vi "Register gRPC Messages.vi"(8 "error in (no error)":errorcluster, 11 "gRPC ID":T1) -> (0 "error out":errorcluster, 3 "gRPC ID Out":T1)   [LabVIEW 2021, in "NI Switch Client.lvlib"]
uses:
  NI Switch Client.lvlib
  <vilib>/gRPC/LabVIEW gRPC Library/Shared/grpcId.ctl
  <vilib>/gRPC/LabVIEW gRPC Library/Server API/typeDefs/Message Metadata.ctl
  <vilib>/gRPC/LabVIEW gRPC Library/Server API/typeDefs/Message Element Metadata.ctl
  <vilib>/gRPC/LabVIEW gRPC Library/Server API/typeDefs/Message Element Type.ctl
  <vilib>/gRPC/LabVIEW gRPC Library/Server API/typeDefs/Enum Metadata.ctl
  <vilib>/gRPC/LabVIEW gRPC Library/grpc-lvsupport-release.lvlib
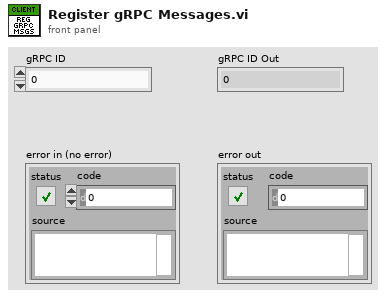
[diagram p1: front panel]
types:
  T1 = typedef "grpc-lvsupport-release.lvlib/grpcId.ctl" = u64
  T2 = typedef "grpc-lvsupport-release.lvlib/Enum Metadata.ctl" = cluster{"Version":i32, "Name":string, "Type Url":string, "Enum Values":string, "Allow Alias":bool}
  T3 = typedef "grpc-lvsupport-release.lvlib/Message Metadata.ctl" = cluster{"Version":i32, "Name":string, "Type Url":string, "Elements":T4[], "Has Oneof":bool}
  T4 = typedef "grpc-lvsupport-release.lvlib/Message Element Metadata.ctl" = cluster{"Field Name":string, "Embedded Message Name":string, "Protobuf Index":i32, "MessageElementType":T5, "Repeated":bool, "Is in Oneof":bool, "Oneof Container Name":string}
  T5 = typedef "grpc-lvsupport-release.lvlib/Message Element Type.ctl" = enum32{"Int32Value", "FloatValue", "DoubleValue", "BoolValue", "StringValue", "MessageValue", "Int64Value", "UInt32Value", "UInt64Value", "EnumValue", "Bytes", "Fixed64", "Fixed32", "SFixed64", "SFixed32", "SInt64", "SInt32"}
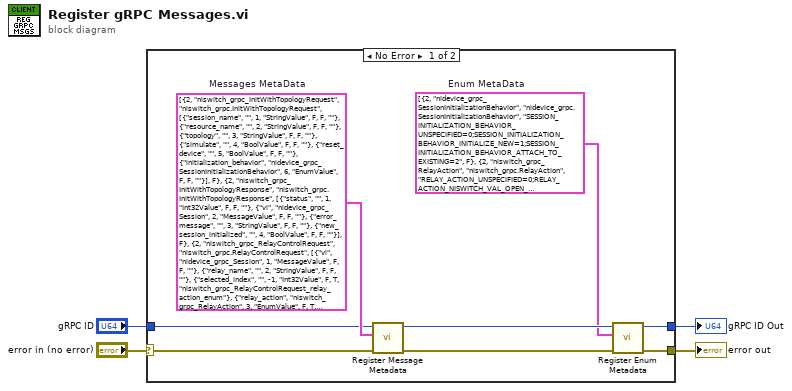
[diagram p0: block diagram]
diagram:
  n1 = case shown="No Error" "error in (no error)" {
    selector: "error in (no error)" -> [w10 w13]
    tunnel: [w9 w12] -> w1
    tunnel: [w6 w13] -> w4
    tunnel: "gRPC ID" -> [w9 w12]
    frame No Error {
      w5 = T2[] [{"Version"=2, "Name"="nidevice_grpc_SessionInitializationBehavior", "Type Url"="nidevice_grpc.SessionInitializationBehavior", "Enum Values"="SESSION_INITIALIZATION_BEHAVIOR_UNSPECIFIED=0;SESSION_INITIALIZATION_BEHAVIOR_INITIALIZE_NEW=1;SESSION_INITIALIZATION_BEHAVIOR_ATTACH_TO_EXISTING=2", "Allow Alias"=FALSE}, {"Version"=2, "Name"="niswitch_grpc_RelayAction", "Type Url"="niswitch_grpc.RelayAction", "Enum Values"="RELAY_ACTION_UNSPECIFIED=0;RELAY_ACTION_NISWITCH_VAL_OPEN_RELAY=20;RELAY_ACTION_NISWITCH_VAL_CLOSE_RELAY=21", "Allow Alias"=FALSE}, {"Version"=2, "Name"="niswitch_grpc_RelayPosition", "Type Url"="niswitch_grpc.RelayPosition", "Enum Values"="RELAY_POSITION_UNSPECIFIED=0;RELAY_POSITION_NISWITCH_VAL_OPEN=10;RELAY_POSITION_NISWITCH_VAL_CLOSED=11", "Allow Alias"=FALSE}]  # Enum MetaData
      w11 = T3[] [{"Version"=2, "Name"="niswitch_grpc_InitWithTopologyRequest", "Type Url"="niswitch_grpc.InitWithTopologyRequest", "Elements"=[{"Field Name"="session_name", "Embedded Message Name"="", "Protobuf Index"=1, "MessageElementType"=enum."StringValue", "Repeated"=FALSE, "Is in Oneof"=FALSE, "Oneof Container Name"=""}, {"Field Name"="resource_name", "Embedded Message Name"="", "Protobuf Index"=2, "MessageElementType"=enum."StringValue", "Repeated"=FALSE, "Is in Oneof"=FALSE, "Oneof Container Name"=""}, {"Field Name"="topology", "Embedded Message Name"="", "Protobuf Index"=3, "MessageElementType"=enum."StringValue", "Repeated"=FALSE, "Is in Oneof"=FALSE, "Oneof Container Name"=""}, {"Field Name"="simulate", "Embedded Message Name"="", "Protobuf Index"=4, "MessageElementType"=enum."BoolValue", "Repeated"=FALSE, "Is in Oneof"=FALSE, "Oneof Container Name"=""}, {"Field Name"="reset_device", "Embedded Message Name"="", "Protobuf Index"=5, "MessageElementType"=enum."BoolValue", "Repeated"=FALSE, "Is in Oneof"=FALSE, "Oneof Container Name"=""}, {"Field Name"="initialization_behavior", "Embedded Message Name"="nidevice_grpc_SessionInitializationBehavior", "Protobuf Index"=6, "MessageElementType"=enum."EnumValue", "Repeated"=FALSE, "Is in Oneof"=FALSE, "Oneof Container Name"=""}], "Has Oneof"=FALSE}, {"Version"=2, "Name"="niswitch_grpc_InitWithTopologyResponse", "Type Url"="niswitch_grpc.InitWithTopologyResponse", "Elements"=[{"Field Name"="status", "Embedded Message Name"="", "Protobuf Index"=1, "MessageElementType"=enum."Int32Value", "Repeated"=FALSE, "Is in Oneof"=FALSE, "Oneof Container Name"=""}, {"Field Name"="vi", "Embedded Message Name"="nidevice_grpc_Session", "Protobuf Index"=2, "MessageElementType"=enum."MessageValue", "Repeated"=FALSE, "Is in Oneof"=FALSE, "Oneof Container Name"=""}, {"Field Name"="error_message", "Embedded Message Name"="", "Protobuf Index"=3, "MessageElementType"=enum."StringValue", "Repeated"=FALSE, "Is in Oneof"=FALSE, "Oneof Container Name"=""}, {"Field Name"="new_session_initialized", "Embedded Message Name"="", "Protobuf Index"=4, "MessageElementType"=enum."BoolValue", "Repeated"=FALSE, "Is in Oneof"=FALSE, "Oneof Container Name"=""}], "Has Oneof"=FALSE}, {"Version"=2, "Name"="niswitch_grpc_RelayControlRequest", "Type Url"="niswitch_grpc.RelayControlRequest", "Elements"=[{"Field Name"="vi", "Embedded Message Name"="nidevice_grpc_Session", "Protobuf Index"=1, "MessageElementType"=enum."MessageValue", "Repeated"=FALSE, "Is in Oneof"=FALSE, "Oneof Container Name"=""}, {"Field Name"="relay_name", "Embedded Message Name"="", "Protobuf Index"=2, "MessageElementType"=enum."StringValue", "Repeated"=FALSE, "Is in Oneof"=FALSE, "Oneof Container Name"=""}, {"Field Name"="selected_index", "Embedded Message Name"="", "Protobuf Index"=-1, "MessageElementType"=enum."Int32Value", "Repeated"=FALSE, "Is in Oneof"=TRUE, "Oneof Container Name"="niswitch_grpc_RelayControlRequest_relay_action_enum"}, {"Field Name"="relay_action", "Embedded Message Name"="niswitch_grpc_RelayAction", "Protobuf Index"=3, "MessageElementType"=enum."EnumValue", "Repeated"=FALSE, "Is in Oneof"=TRUE, "Oneof Container Name"="niswitch_grpc_RelayControlRequest_relay_action_enum"}, {"Field Name"="relay_action_raw", "Embedded Message Name"="", "Protobuf Index"=4, "MessageElementType"=enum."SInt32", "Repeated"=FALSE, "Is in Oneof"=TRUE, "Oneof Container Name"="niswitch_grpc_RelayControlRequest_relay_action_enum"}], "Has Oneof"=TRUE}, {"Version"=2, "Name"="niswitch_grpc_RelayControlResponse", "Type Url"="niswitch_grpc.RelayControlResponse", "Elements"=[{"Field Name"="status", "Embedded Message Name"="", "Protobuf Index"=1, "MessageElementType"=enum."Int32Value", "Repeated"=FALSE, "Is in Oneof"=FALSE, "Oneof Container Name"=""}], "Has Oneof"=FALSE}, {"Version"=2, "Name"="niswitch_grpc_GetRelayPositionRequest", "Type Url"="niswitch_grpc.GetRelayPositionRequest", "Elements"=[{"Field Name"="vi", "Embedded Message Name"="nidevice_grpc_Session", "Protobuf Index"=1, "MessageElementType"=enum."MessageValue", "Repeated"=FALSE, "Is in Oneof"=FALSE, "Oneof Container Name"=""}, {"Field Name"="relay_name", "Embedded Message Name"="", "Protobuf Index"=2, "MessageElementType"=enum."StringValue", "Repeated"=FALSE, "Is in Oneof"=FALSE, "Oneof Container Name"=""}], "Has Oneof"=FALSE}, {"Version"=2, "Name"="niswitch_grpc_GetRelayPositionResponse", "Type Url"="niswitch_grpc.GetRelayPositionResponse", "Elements"=[{"Field Name"="status", "Embedded Message Name"="", "Protobuf Index"=1, "MessageElementType"=enum."Int32Value", "Repeated"=FALSE, "Is in Oneof"=FALSE, "Oneof Container Name"=""}, {"Field Name"="relay_position", "Embedded Message Name"="niswitch_grpc_RelayPosition", "Protobuf Index"=2, "MessageElementType"=enum."EnumValue", "Repeated"=FALSE, "Is in Oneof"=FALSE, "Oneof Container Name"=""}, {"Field Name"="relay_position_raw", "Embedded Message Name"="", "Protobuf Index"=3, "MessageElementType"=enum."SInt32", "Repeated"=FALSE, "Is in Oneof"=FALSE, "Oneof Container Name"=""}], "Has Oneof"=FALSE}, {"Version"=2, "Name"="niswitch_grpc_WaitForDebounceRequest", "Type Url"="niswitch_grpc.WaitForDebounceRequest", "Elements"=[{"Field Name"="vi", "Embedded Message Name"="nidevice_grpc_Session", "Protobuf Index"=1, "MessageElementType"=enum."MessageValue", "Repeated"=FALSE, "Is in Oneof"=FALSE, "Oneof Container Name"=""}, {"Field Name"="maximum_time_ms", "Embedded Message Name"="", "Protobuf Index"=2, "MessageElementType"=enum."SInt32", "Repeated"=FALSE, "Is in Oneof"=FALSE, "Oneof Container Name"=""}], "Has Oneof"=FALSE}, {"Version"=2, "Name"="niswitch_grpc_WaitForDebounceResponse", "Type Url"="niswitch_grpc.WaitForDebounceResponse", "Elements"=[{"Field Name"="status", "Embedded Message Name"="", "Protobuf Index"=1, "MessageElementType"=enum."Int32Value", "Repeated"=FALSE, "Is in Oneof"=FALSE, "Oneof Container Name"=""}], "Has Oneof"=FALSE}, {"Version"=2, "Name"="niswitch_grpc_CloseRequest", "Type Url"="niswitch_grpc.CloseRequest", "Elements"=[{"Field Name"="vi", "Embedded Message Name"="nidevice_grpc_Session", "Protobuf Index"=1, "MessageElementType"=enum."MessageValue", "Repeated"=FALSE, "Is in Oneof"=FALSE, "Oneof Container Name"=""}], "Has Oneof"=FALSE}, {"Version"=2, "Name"="niswitch_grpc_CloseResponse", "Type Url"="niswitch_grpc.CloseResponse", "Elements"=[{"Field Name"="status", "Embedded Message Name"="", "Protobuf Index"=1, "MessageElementType"=enum."Int32Value", "Repeated"=FALSE, "Is in Oneof"=FALSE, "Oneof Container Name"=""}], "Has Oneof"=FALSE}, {"Version"=2, "Name"="nidevice_grpc_Session", "Type Url"="nidevice_grpc.Session", "Elements"=[{"Field Name"="selected_index", "Embedded Message Name"="", "Protobuf Index"=-1, "MessageElementType"=enum."Int32Value", "Repeated"=FALSE, "Is in Oneof"=TRUE, "Oneof Container Name"="nidevice_grpc_Session_session"}, {"Field Name"="name", "Embedded Message Name"="", "Protobuf Index"=1, "MessageElementType"=enum."StringValue", "Repeated"=FALSE, "Is in Oneof"=TRUE, "Oneof Container Name"="nidevice_grpc_Session_session"}, {"Field Name"="id", "Embedded Message Name"="", "Protobuf Index"=2, "MessageElementType"=enum."UInt32Value", "Repeated"=FALSE, "Is in Oneof"=TRUE, "Oneof Container Name"="nidevice_grpc_Session_session"}], "Has Oneof"=TRUE}]  # Messages MetaData
      n2 = call <vilib>:"Register Message Metadata.vi"("error in"=w10, "Messages"=w11, "gRPCid in"=w9) -> ("error out"=w7:errorcluster, "gRPCid out"=w8:T1)  [unwired: 7 in]
      n3 = call <vilib>:"Register Enum Metadata.vi"("error in"=w7, "Enum Metadata"=w5, "gRPCid in"=w8) -> ("error out"=w6:errorcluster)  [unwired: 7 in, 1 out]
    }
    frame Error {
    }
  }
  "error out" <- w4
  "gRPC ID Out" <- w1
